vi "ActionVIOnCompile_InlineAsync.vi"(8 "error in (no error)":errorcluster, 11 "Device Item Ref in":T1 format="%.0x") -> (0 "error out":errorcluster)   [LabVIEW 2020]
uses:
  <vilib>/NI VeriStand/Custom Device API/Custom Device Item Ref.ctl
  <vilib>/NI VeriStand/Custom Device API/Get Item Property (U16).vi
  <vilib>/NI VeriStand/Custom Device Tools/Custom Device Utility Library/NI VeriStand - Search for Item by Name.vi
  <vilib>/NI VeriStand/Custom Device API/Set Item Property (Variant).vi
  <vilib>/NI VeriStand/Custom Device Tools/Custom Device Utility Library/Custom Device Utility Library.lvlib
  <vilib>/NI VeriStand/Custom Device API/Custom Device API.lvlib
  <vilib>/NI/NIVS Inline Async API/_Data Access System Explorer/Data Access System Explorer.lvlib
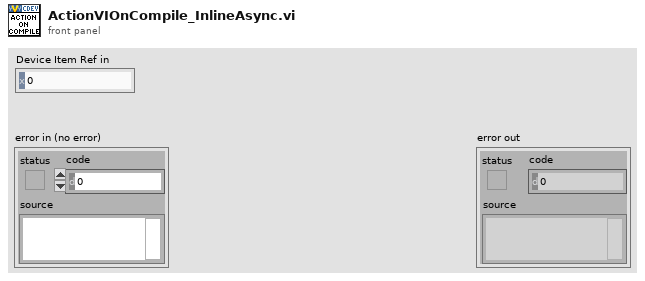
[diagram p1: front panel]
types:
  T1 = typedef "Custom Device API.lvlib/Custom Device Item Ref.ctl" = u64
  T2 = cluster{"Name":string, "Type":enum16{"Output/Write", "Input/Read", "Input/ReadWrite"}, "VS Refs":T1[]}
  T3 = enum16{"Output/Write", "Input/Read", "Input/ReadWrite"}
  T4 = typedef "Custom Device API.lvlib/Custom Device Item Info.ctl" = cluster{"Name":string, "Is Channel":bool, "GUID":string, "Is Waveform":bool}
  T5 = cluster{"Name":string, "Type":enum16{"Output/Write", "Input/Read", "Input/ReadWrite"}, "VS Refs":T1[]}[]
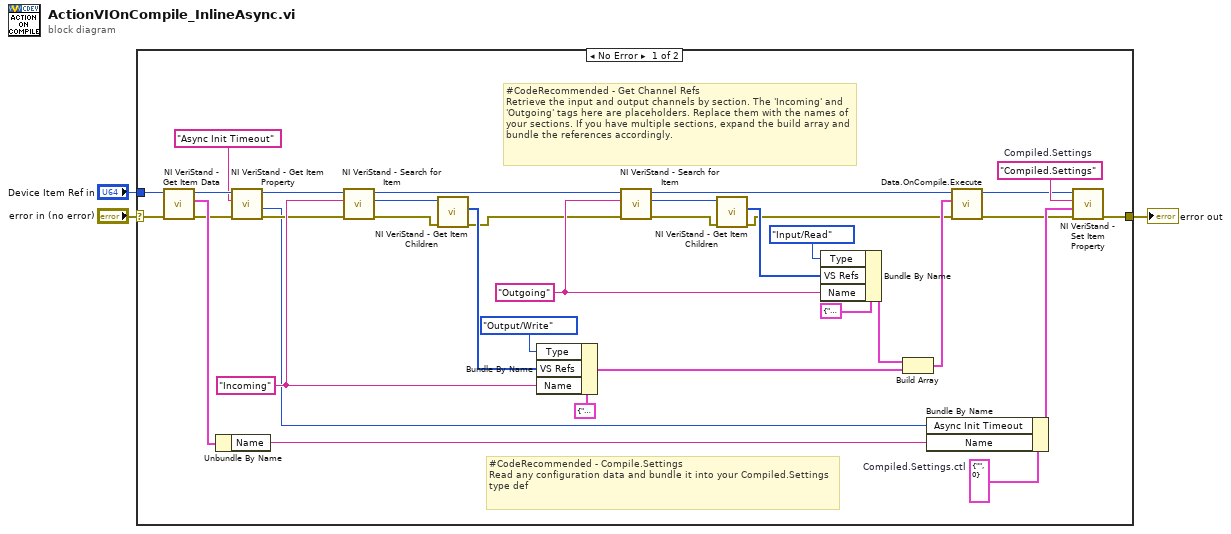
[diagram p0: block diagram]
diagram:
  n1 = case shown="No Error" "error in (no error)" {
    selector: "error in (no error)" -> [w31 w39]
    tunnel: [w32 w39] -> w2
    tunnel: "Device Item Ref in" -> [w30 _]
    frame No Error {
      w10 = cluster{"Name":string, "Async Init Timeout":u16} {"Name"="", "Async Init Timeout"=0}  # Compiled.Settings.ctl
      w25 = "Outgoing" ("Item Name")
      w27 = "Incoming" ("Item Name")
      w34 = "Compiled.Settings"  # Compiled.Settings
      # "#CodeRecommended - Get Channel Refs\nRetrieve the input and output channels by section. The 'Incoming' and 'Outgoing' tags here are placeholders. Replace them with the names of your sections. If you have multiple sections, expand the build array and bundle the references accordingly."
      # "#CodeRecommended - Compile.Settings\nRead any configuration data and bundle it into your Compiled.Settings type def"
      n2 = call <vilib>:"NI VeriStand - Get Item Data.vi"("error in (no error)"=w31, "Item Ref in"=w30) -> ("error out"=w9:errorcluster, "Item Info"=w29:T4, "Item Ref out"=w7:T1)  [unwired: 6 in, 1 out]
      n3 = Unbundle By Name(w29) -> ("Name"=w28:string)
      n4 = call-poly <vilib>:"NI VeriStand - Get Item Property.vi"("error in (no error)"=w9, "Property Name"="Async Init Timeout", "Item Ref in"=w7) -> ("error out"=w8:errorcluster, "Value"=w4:u16, "Item Ref out"=w6:T1)  [unwired: 5 in, 1 out]
      n5 = call-poly <vilib>:"NI VeriStand - Search for Item.vi"("error in"=w8, "Item Name"=w27, "Section Ref in"=w6) -> ("error out"=w38:errorcluster, "Item Ref"=w37:T1, "Section Ref out"=w14:T1)  [unwired: 5 in, 1 out]
      n6 = call <vilib>:"NI VeriStand - Get Item Children.vi"("error in (no error)"=w38, "Item Ref in"=w37) -> ("error out"=w13:errorcluster, "Child Refs"=w26:T1[])  [unwired: 6 in, 2 out]
      n7 = Bundle By Name(cluster=T2 {"Name"="", "Type"=enum."Output/Write", "VS Refs"=[]} ("Group"), "Type"=T3."Output/Write", "VS Refs"=w26, "Name"=w27) -> (w17:T2)
      n8 = call-poly <vilib>:"NI VeriStand - Search for Item.vi"("error in"=w13, "Item Name"=w25, "Section Ref in"=w14) -> ("error out"=w35:errorcluster, "Item Ref"=w36:T1, "Section Ref out"=w15:T1)  [unwired: 5 in, 1 out]
      n9 = call <vilib>:"NI VeriStand - Get Item Children.vi"("error in (no error)"=w35, "Item Ref in"=w36) -> ("error out"=w16:errorcluster, "Child Refs"=w21:T1[])  [unwired: 6 in, 2 out]
      n10 = Bundle By Name(cluster=T2 {"Name"="", "Type"=enum."Output/Write", "VS Refs"=[]} ("Group"), "Type"=T3."Input/Read", "VS Refs"=w21, "Name"=w25) -> (w23:T2)
      n11 = Build Array(w23, w17) -> (w20:T5)
      n12 = Bundle By Name(cluster=w10, "Async Init Timeout"=w4, "Name"=w28) -> (w33:cluster{"Name":string, "Async Init Timeout":u16})
      n13 = call <vilib>:"Data.OnCompile.Execute.vi"("error in"=w16, "VS Ref Groups"=w20, "Custom Device Ref"=w15) -> ("error out"=w12:errorcluster, "Custom Device Ref"=w11:T1)  [unwired: 7 in]
      n14 = call-poly <vilib>:"NI VeriStand - Set Item Property.vi"("error in (no error)"=w12, "Value"=w33, "Property Name"=w34, "Item Ref in"=w11) -> ("error out"=w32:errorcluster)  [unwired: 5 in, 2 out]
    }
    frame Error {
    }
  }
  "error out" <- w2
